vi "02WRITE REG.vi"(3 "Password":string="\u0003\u0002\u0001\u0000", 4 "Nombre":string="LabVIEW") -> ()   [LabVIEW 2010]
uses:
  <vilib>/registry/registry.llb/Registry RtKey.ctl
  <vilib>/registry/registry.llb/Write Registry Value Simple.vi
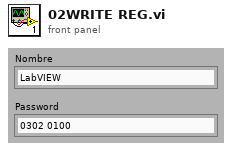
[diagram p1: front panel]
types:
  T1 = typedef "Registry RtKey.ctl" = enum32{"HKEY_CLASSES_ROOT", "HKEY_CURRENT_USER", "HKEY_LOCAL_MACHINE", "HKEY_USERS", "HKEY_PERFORMANCE_DATA", "HKEY_CURRENT_CONFIG", "HKEY_DYN_DATA"}
  T2 = typedef "Registry refnum.ctl" = refnum<k1>
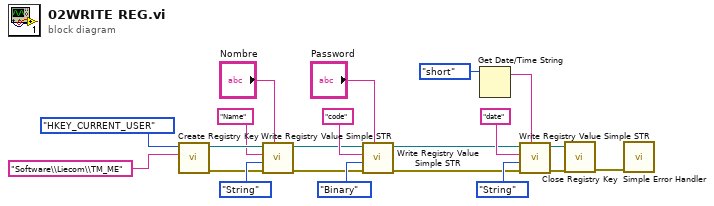
[diagram p0: block diagram]
diagram:
  n1 = call <vilib>:"Create Registry Key.vi"("subkey"="Software\\Liecom\\TM_ME", "root key (HKEY_LOCAL_MACHINE)"=Registry_RtKey."HKEY_CURRENT_USER") -> ("error out"=w15:errorcluster, "refnum out"=w19:T2)  [unwired: 7 in, 1 out]
  n2 = call-poly <vilib>:"Write Registry Value Simple STR.vi"("String/Binary data"="Nombre", "error in (no error)"=w15, "simple data type"=enum16{"String", "Binary", "DWORD"}."String", "value"="Name", "refnum"=w19) -> ("error out"=w9:errorcluster, "refnum out"=w10:T2)  [unwired: 3 in]
  n3 = call-poly <vilib>:"Write Registry Value Simple STR.vi"("String/Binary data"="Password", "error in (no error)"=w9, "simple data type"=enum16{"String", "Binary", "DWORD"}."Binary", "value"="code", "refnum"=w10) -> ("error out"=w4:errorcluster, "refnum out"=w5:T2)  [unwired: 3 in]
  n4 = Get Date/Time String(date format (0)=enum16{"short", "long", "abbreviated"}."short") -> (date string=w3:string)  [unwired: 2 in, 1 out]
  n5 = call-poly <vilib>:"Write Registry Value Simple STR.vi"("String/Binary data"=w3, "error in (no error)"=w4, "simple data type"=enum16{"String", "Binary", "DWORD"}."String", "value"="date", "refnum"=w5) -> ("error out"=w1:errorcluster, "refnum out"=w2:T2)  [unwired: 3 in]
  n6 = call <vilib>:"Close Registry Key.vi"("error in (no error)"=w1, "refnum"=w2) -> ("error out"=w20:errorcluster)  [unwired: 5 in]
  n7 = call <vilib>:"Simple Error Handler.vi"("error in (no error)"=w20) -> ()  [unwired: 4 in, 5 out]
